vi "Stock Data - Download.vi"(8 "error in":errorcluster, 11 "URL":string) -> (0 "error out":errorcluster, 2 "headers":string, 3 "Raw Stock Data":string)   [LabVIEW 2011]
doc: "Download Stock Data from URL using HTTP.\n\nInputs:\n URL: \n Error in: Error cluster\n\nOutputs:\n Header: HTTP header.\n Raw Stock Data: This is the body of the HTTP request.\n Error out: Error cluster"
uses:
  <vilib>/httpClient/LabVIEWHTTPClient.lvlib
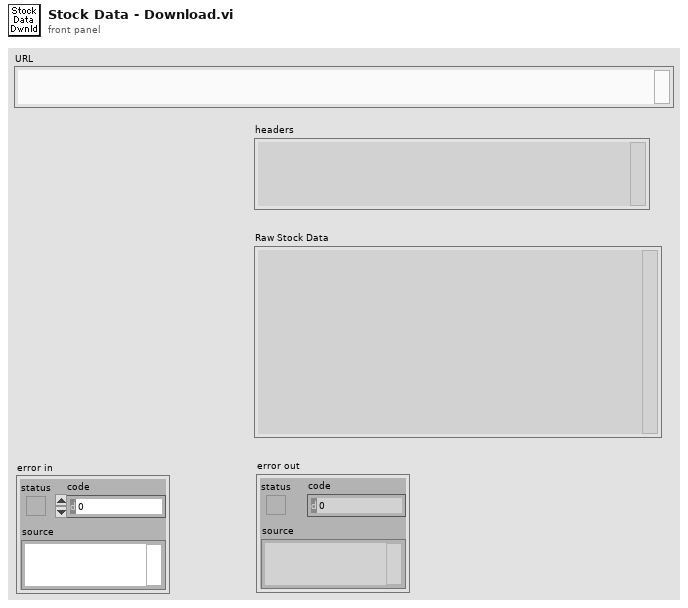
[diagram p1: front panel]
types:
  T1 = typedef "LabVIEWHTTPClient.lvlib/ClientHandle.ctl" = refnum<k1>
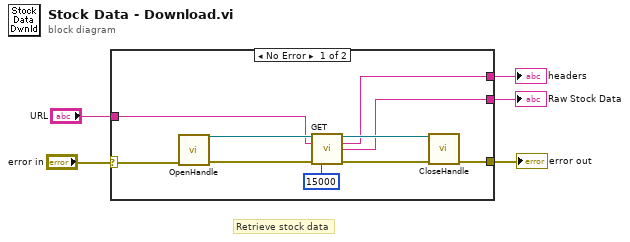
[diagram p0: block diagram]
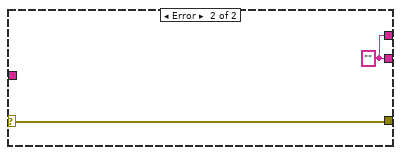
[diagram p2: hidden frame]
diagram:
  # "Retrieve stock data"
  n1 = case shown="No Error" "error in" {
    selector: "error in" -> [w7 w17]
    tunnel: "URL" -> [w13 _]
    tunnel: [w10 w16] -> w4
    tunnel: [w9 w16] -> w3
    tunnel: [w8 w17] -> w2
    frame No Error {
      n2 = call <vilib>:"OpenHandle.vi"("error in (no error)"=w7) -> ("client handle out"=w15:T1, "error out"=w14:errorcluster)  [unwired: 13 in]
      n3 = call <vilib>:"GET.vi"("client handle"=w15, "url"=w13, "error in (no error)"=w14, "timeout (10000)"=15000) -> ("client handle out"=w12:T1, "headers"=w9:string, "body"=w10:string, "error out"=w11:errorcluster)  [unwired: 8 in]
      n4 = call <vilib>:"CloseHandle.vi"("client handle"=w12, "error in (no error)"=w11) -> ("error out"=w8:errorcluster)  [unwired: 13 in]
    }
    frame Error {
      w16 = "" ("body")
    }
  }
  "Raw Stock Data" <- w4
  "headers" <- w3
  "error out" <- w2
